vi "Read Cycling Count.vi"(8 "error in (no error)":errorcluster, 11 "VISA resource name":refnum<visa-resource-name>) -> (0 "error out":errorcluster, 1 "Cycling Count":dbl, 3 "VISA resource name out":refnum<visa-resource-name>)   [LabVIEW 2012, in "Temptronic TP04300.lvlib"]
doc: "This VI reads the current cycle number if cycling, the last value if not. \n\nNote: If Version 1 compatibility mode is enabled, this function returns the number of fully completed cycles."
uses:
  <instrlib>/Temptronic TP04300/Temptronic TP04300.lvlib
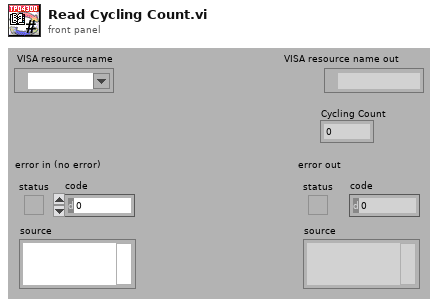
[diagram p1: front panel]
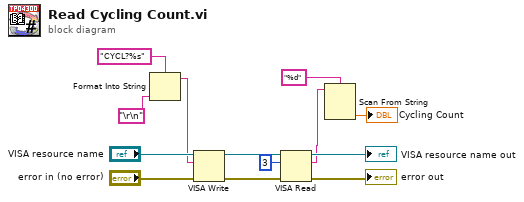
[diagram p0: block diagram]
diagram:
  n1 = Format Into String(format string="CYCL?%s", "\r\n") -> (resulting string=w10:string)  [unwired: 2 in, 1 out]
  n2 = VISA Write(VISA resource name="VISA resource name", write buffer=w10, error in (no error)="error in (no error)") -> (VISA resource name out=w8:refnum<visa-resource-name>, error out=w6:errorcluster)  [unwired: 1 out]
  n3 = VISA Read(VISA resource name=w8, byte count=u32 3, error in (no error)=w6) -> (VISA resource name out=→"VISA resource name out":refnum<visa-resource-name>, read buffer=w1:string, error out=→"error out":errorcluster)  [unwired: 1 out]
  n4 = Scan From String(format string="%d", input string=w1) -> (output 1=→"Cycling Count":dbl)  [unwired: 3 in, 3 out]
